vi "Read Event Class.vi"(2 "Enclave":T1) -> (7 "Event":refnum<class "Event.lvclass">, 9 "error out":errorcluster)   [LabVIEW 2022 SP3, in "Enclave.lvlib"]
doc: "Generates a class instance that wraps an event based reader. An event registration can be created by the class to be used with dynamic event terminals. Note that events are less efficient than lossless readers and are intended for lower rate data/messages.\n\nThe event is registered before the event reader class is returned and will be able to handle any events after this VI is called, therefore the reader should not be created long before the event structure runs to prevent excessive enqueuing of events to be handled if data is already being written."
uses:
  Enclave.lvlib
  ))Channel.ctl
  Element.ctl
  Event/Event.lvclass
  Operation.ctl
  Enclave/Enclave.lvclass
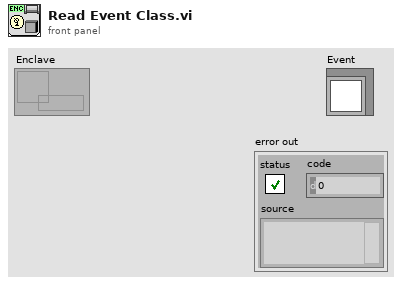
[diagram p1: front panel]
types:
  T1 = typedef "Enclave.lvlib/))Channel.ctl" = refnum<queue>
  T2 = typedef "Enclave.lvlib/Operation.ctl" = enum16{"Get Core", "Init", "Close"}
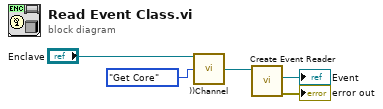
[diagram p0: block diagram]
diagram:
  n1 = call "))Channel.vi"("EnclaveChannel in"="Enclave", "Operation"=Operation."Get Core") -> ("Enclave"=w4:refnum<class "Enclave.lvclass">)  [unwired: 11 in, 2 out]
  n2 = call "Create Event Reader.vi"("Enclave in"=w4) -> ("error out"=→"error out":errorcluster, "Event"=→"Event":refnum<class "Event.lvclass">)  [unwired: 8 in, 1 out]
